vi "CalculateGap.vi"(0 "object in":refnum<class "PenaltyTactic.lvclass">, 2 "factor":dbl, 3 "FieldRef":refnum<class "Field.lvclass">, 5 "error in (no error)":errorcluster) -> (14 "object out":refnum<class "PenaltyTactic.lvclass">, 16 "gap":dbl[](array[numeric]), 19 "error out":errorcluster)   [LabVIEW 2023, in "PenaltyTactic.lvclass"]
uses:
  PenaltyTactic.lvclass
  Field_class/Field.lvclass
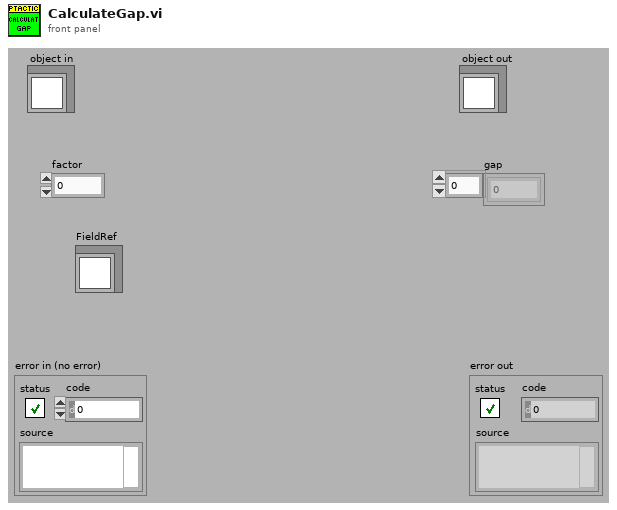
[diagram p1: front panel]
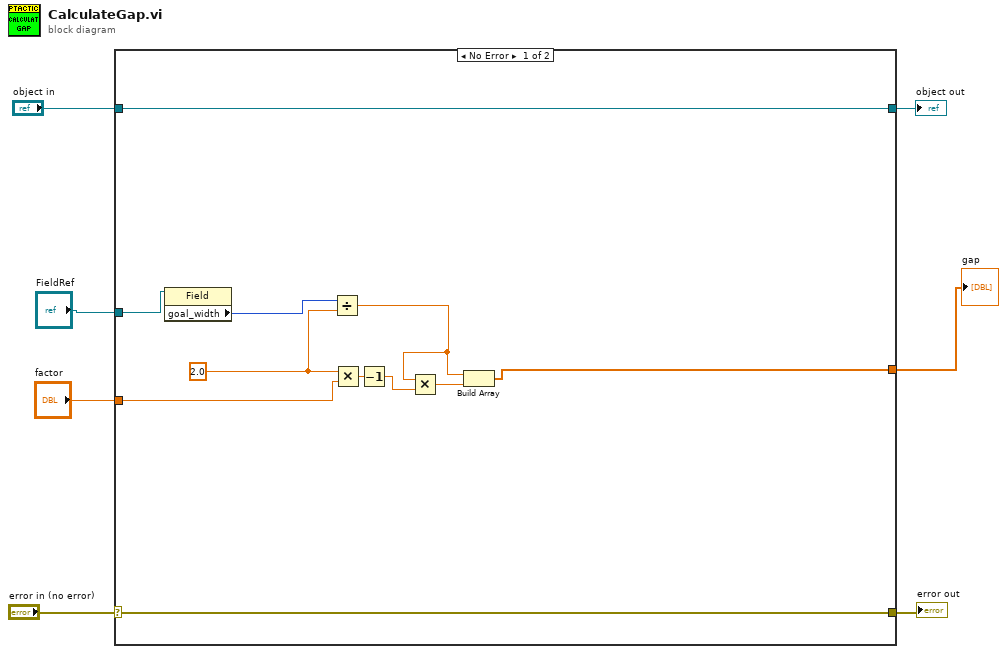
[diagram p0: block diagram]
diagram:
  n1 = case shown="No Error" "error in (no error)" {
    selector: "error in (no error)" -> [w18 w20]
    tunnel: [w18 w20] -> w6
    tunnel: [w17 w19] -> w4
    tunnel: "object in" -> [w17 w19]
    tunnel: "factor" -> [w14 _]
    tunnel: "FieldRef" -> [w13 _]
    tunnel: [w8 _] -> w1
    frame No Error {
      w11 = 2.0 ("x")
      n2 = property class="Field"(reference=w13) -> ("goal_width"=w12:i32)  [unwired: 1 in, 2 out]
      n3 = Divide(x=w12, y=w11) -> (x/y=w9:dbl)
      n4 = Multiply(x=w11, y=w14) -> (x*y=w15:dbl)
      n5 = Decrement(x=w15) -> (x-1=w10:dbl)
      n6 = Multiply(x=w9, y=w10) -> (x*y=w16:dbl)
      n7 = Build Array(w9, w16) -> (w8:dbl[])
    }
    frame Error {
    }
  }
  "error out" <- w6
  "object out" <- w4
  "gap" <- w1
